vi "tpg361_get_status.vi"(5 "tpg361_delay 3":u32=500, 6 "tpg361_delay 2":u32=500, 7 "err_in":errorcluster, 8 "tpg361_delay":u32=500, 10 "tpg361_visa":refnum<visa-resource-name>) -> (0 "err_out":errorcluster, 3 "Gauge status":bool)   [LabVIEW 2019]
panel:
  out "Overall Status":bool
  out "Acknowledgement Status":bool
  out "tpg361_visa 2":refnum<visa-resource-name>
  in  "tpg361_b2r 2":u32
  in  "tpg361_b2r":u32
  # "VISA"
  # "DELAY"
  # "BYTE AT PORT"
  # "STATUS"
  # "ERROR"
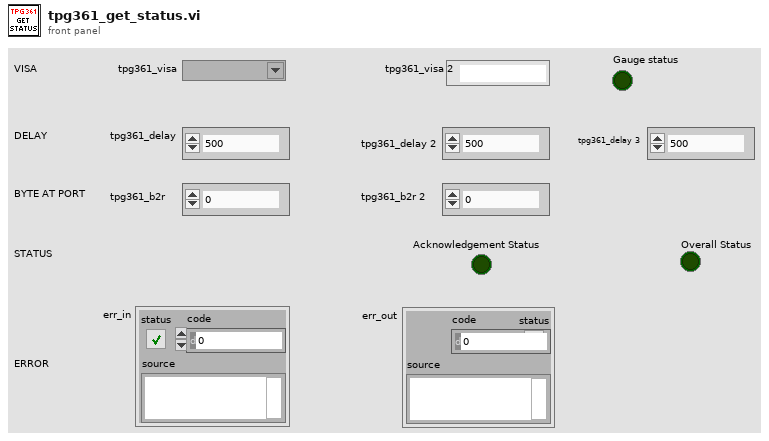
[diagram p1: front panel]
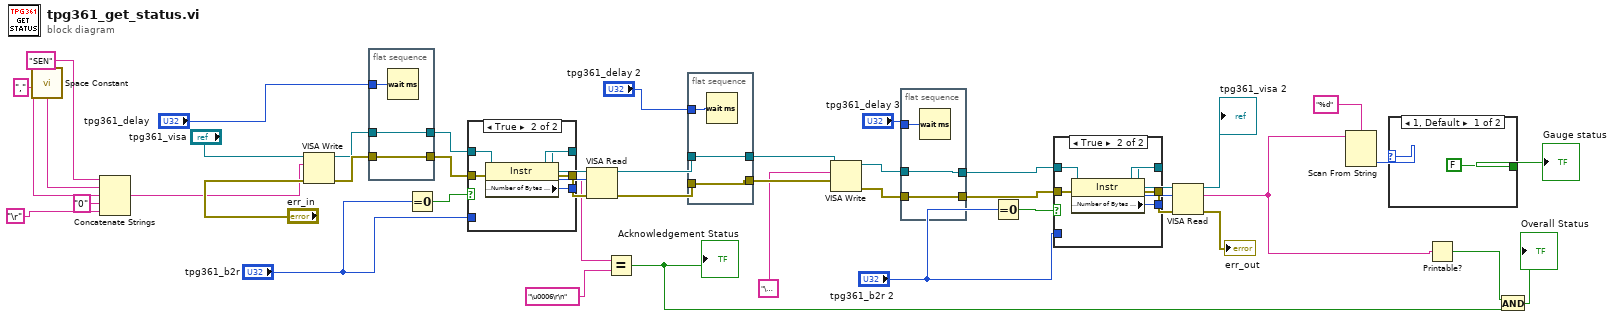
[diagram p0: block diagram]
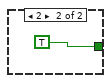
[diagram p2: hidden frame]
diagram:
  n1 = call <vilib>:"Space Constant.vi"() -> ("String"=w8:string)
  n2 = Concatenate Strings("SEN" ("string"), w8, "," ("string"), "0" ("string"), "\r") -> (w17:string)
  n3 = VISA Write(VISA resource name="tpg361_visa", write buffer=w17, error in (no error)="err_in") -> (VISA resource name out=w43:refnum<visa-resource-name>, error out=w45:errorcluster)  [unwired: 1 out]
  n4 = flat-sequence {
    tunnel: w45 -> [w47]
    tunnel: [w47] -> w44
    tunnel: w43 -> [w46]
    tunnel: [w46] -> w42
    tunnel: "tpg361_delay" -> [w48]
    frame #0 {
      n5 = Wait (ms)(milliseconds to wait=w48) -> ()  [unwired: 1 out]
    }
  }
  n6 = Equal To 0?(x="tpg361_b2r") -> (x = 0?=w38:bool)
  n7 = case shown="True" w38 {
    tunnel: w44 -> [w50 w56]
    tunnel: w42 -> [w51 w55]
    tunnel: [w51 w54] -> w36
    tunnel: [w50 w53] -> w35
    tunnel: [w49 w52] -> w34
    tunnel: "tpg361_b2r" -> [w49 _]
    frame False {
    }
    frame True {
      n8 = property class="Instr"(reference=w55, error in=w56) -> (reference out=w54:refnum<visa-resource-name>, error out=w53:errorcluster, "Serial Settings:Number of Bytes at Serial Port"=w52:u32)
    }
  }
  n9 = VISA Read(VISA resource name=w36, byte count=w34, error in (no error)=w35) -> (VISA resource name out=w33:refnum<visa-resource-name>, read buffer=w15:string, error out=w32:errorcluster)  [unwired: 1 out]
  n10 = Equal?(x=w15, y="\u0006\r\n") -> (x = y?=w11:bool)
  "Acknowledgement Status" <- w11
  n11 = flat-sequence {
    tunnel: [w57] -> w30
    tunnel: w33 -> [w59]
    tunnel: [w59] -> w31
    tunnel: "tpg361_delay 2" -> [w58]
    tunnel: w32 -> [w57]
    frame #0 {
      n12 = Wait (ms)(milliseconds to wait=w58) -> ()  [unwired: 1 out]
    }
  }
  n13 = VISA Write(VISA resource name=w31, write buffer="\u0005", error in (no error)=w30) -> (VISA resource name out=w23:refnum<visa-resource-name>, error out=w22:errorcluster)  [unwired: 1 out]
  n14 = flat-sequence {
    tunnel: [w61] -> w29
    tunnel: [w62] -> w28
    tunnel: w23 -> [w62]
    tunnel: w22 -> [w61]
    tunnel: "tpg361_delay 3" -> [w60]
    frame #0 {
      n15 = Wait (ms)(milliseconds to wait=w60) -> ()  [unwired: 1 out]
    }
  }
  n16 = Equal To 0?(x="tpg361_b2r 2") -> (x = 0?=w27:bool)
  n17 = case shown="True" w27 {
    tunnel: w29 -> [w64 w70]
    tunnel: w28 -> [w65 w69]
    tunnel: [w65 w68] -> w26
    tunnel: [w64 w67] -> w25
    tunnel: [w63 w66] -> w24
    tunnel: "tpg361_b2r 2" -> [w63 _]
    frame False {
    }
    frame True {
      n18 = property class="Instr"(reference=w69, error in=w70) -> (reference out=w68:refnum<visa-resource-name>, error out=w67:errorcluster, "Serial Settings:Number of Bytes at Serial Port"=w66:u32)
    }
  }
  n19 = VISA Read(VISA resource name=w26, byte count=w24, error in (no error)=w25) -> (VISA resource name out=→"tpg361_visa 2":refnum<visa-resource-name>, read buffer=w3:string, error out=→"err_out":errorcluster)  [unwired: 1 out]
  n20 = Scan From String(format string="%d", input string=w3) -> (output 1=w1:i32)  [unwired: 3 in, 3 out]
  n21 = case shown="1, Default" w1 {
    tunnel: [FALSE TRUE] -> w4
    frame 1, Default {
    }
    frame 2 {
    }
  }
  "Gauge status" <- w4
  n22 = Printable?(1:w3) -> (0:w9:bool)
  n23 = And(x=w9, y=w11) -> (x .and. y?=→"Overall Status":bool)
